vi "close shutter.vi"(8 "error in (no error)":errorcluster, 11 "StageSPIM in":refnum<class "StageSPIM.lvclass">) -> (0 "error out":errorcluster, 3 "StageSPIM out":refnum<class "StageSPIM.lvclass">)   [LabVIEW 2012, in "StageSPIM.lvclass"]
uses:
  StageSPIM.lvclass
  <vilib>/Distrio/Murmex/GenericMessage/GenericMessage.lvclass
  <vilib>/Distrio/Murmex/Message/Add or replace parameter.vi
  <vilib>/Distrio/Murmex/Murmex/Murmex.lvclass
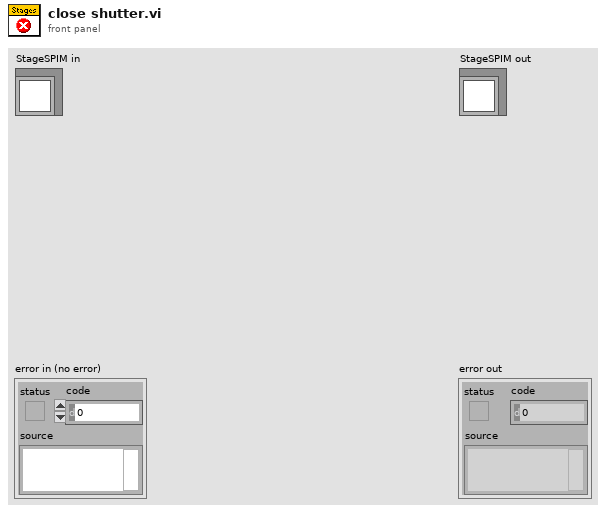
[diagram p1: front panel]
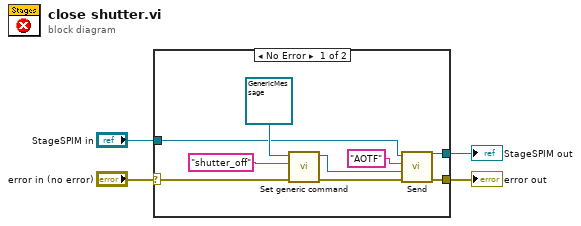
[diagram p0: block diagram]
diagram:
  n1 = case shown="No Error" "error in (no error)" {
    selector: "error in (no error)" -> [w10 w15]
    tunnel: [w9 w15] -> w3
    tunnel: [w5 w14] -> w1
    tunnel: "StageSPIM in" -> [w6 w14]
    frame No Error {
      n2 = call <vilib>:"Set generic command.vi"("error in (no error)"=w10, "generic command"="shutter_off", "GenericMessage in"=refnum<class "GenericMessage.lvclass"> refnum ("Distrio Murmex 1.1:GenericMessage")) -> ("error out"=w11:errorcluster, "GenericMessage out"=w8:refnum<class "GenericMessage.lvclass">)  [unwired: 7 in]
      n3 = call <vilib>:"Send.vi"("error in (no error)"=w11, "Message"=w8, "recipient"="AOTF", "Murmex in"=w6) -> ("error out"=w9:errorcluster, "Murmex out"=w5:refnum<class "StageSPIM.lvclass">)  [unwired: 6 in]
    }
    frame Error {
    }
  }
  "error out" <- w3
  "StageSPIM out" <- w1
